vi "Parse.vi"(8 "error in (no error)":errorcluster, 11 "Array":string[](array[string])) -> (0 "error out":errorcluster, 3 "Double":dbl[](array[numeric]))   [LabVIEW 2018, in "Serial.lvclass"]
uses:
  Serial.lvclass
  5dd0743a-6fd2-4afc-819b-2e410fbb0d41.vi
  S1/S1.lvclass
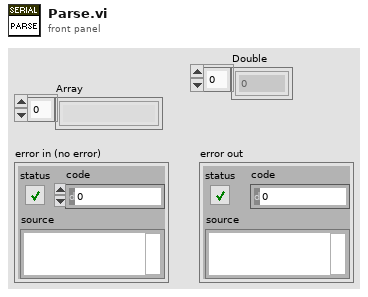
[diagram p1: front panel]
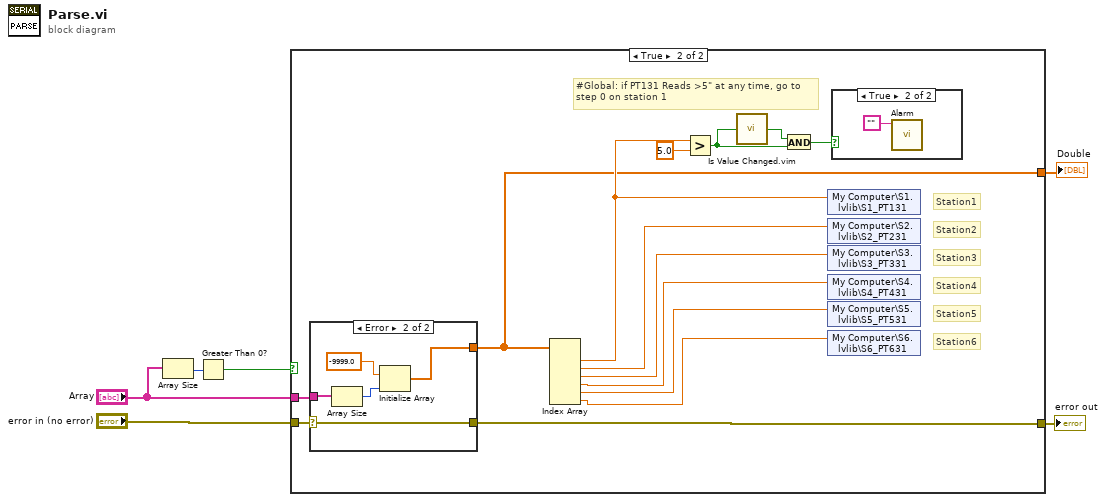
[diagram p0: block diagram]
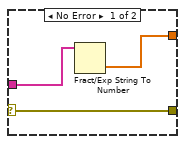
[diagram p4: hidden frame]
diagram:
  n1 = Array Size(array="Array") -> (size(s)=w3:i32)
  n2 = Greater Than 0?(x=w3) -> (x > 0?=w2:bool)
  n3 = case shown="True" w2 {
    tunnel: [w7 w21] -> w6
    tunnel: "error in (no error)" -> [w7 w20]
    tunnel: "Array" -> [_ w19]
    tunnel: [_ w12] -> w1
    frame False {
    }
    frame True {
      # "Station6"
      # "Station5"
      # "Station4"
      # "Station3"
      # "#Global: if PT131 Reads >5\" at any time, go to\nstep 0 on station 1"
      # "Station2"
      # "Station1"
      n4 = case shown="Error" w20 {
        selector: w20 -> [w25 w30]
        tunnel: w19 -> [w24 w28]
        tunnel: [w25 w30] -> w21
        tunnel: [w23 w26] -> w12
        frame No Error {
          n5 = Fract/Exp String To Number(string=w24) -> (number=w23:dbl[])  [unwired: 3 in, 1 out]
        }
        frame Error {
          n6 = Array Size(array=w28) -> (size(s)=w27:i32)
          n7 = Initialize Array(-9999.0 ("element"), w27) -> (w26:dbl[])
        }
      }
      n8 = Index Array(array=w12) -> (element #1=w18:dbl, element #2=w13:dbl, element #3=w11:dbl, element #4=w10:dbl, element #5=w9:dbl, element #6=w8:dbl)  [unwired: 6 in]
      n9 = Greater?(x=w18, y=5.0) -> (0:w15:bool)
      n10 = call "Is Value Changed.vim"("value"=w15) -> ("changed or first call?"=w16:bool)
      n11 = And(x=w16, y=w15) -> (x .and. y?=w14:bool)
      n12 = shared-variable "My Computer\\S1.lvlib\\S1_PT131"(w18) -> ()  [unwired: 1 in, 1 out]
      n13 = shared-variable "My Computer\\S2.lvlib\\S2_PT231"(w13) -> ()  [unwired: 1 in, 1 out]
      n14 = shared-variable "My Computer\\S3.lvlib\\S3_PT331"(w11) -> ()  [unwired: 1 in, 1 out]
      n15 = shared-variable "My Computer\\S4.lvlib\\S4_PT431"(w10) -> ()  [unwired: 1 in, 1 out]
      n16 = shared-variable "My Computer\\S5.lvlib\\S5_PT531"(w9) -> ()  [unwired: 1 in, 1 out]
      n17 = shared-variable "My Computer\\S6.lvlib\\S6_PT631"(w8) -> ()  [unwired: 1 in, 1 out]
      n18 = case shown="True" w14 {
        frame False {
        }
        frame True {
          n19 = call "Alarm.vi"("Alarm"="") -> ()  [unwired: 10 in, 1 out]
        }
      }
    }
  }
  "error out" <- w6
  "Double" <- w1
